vi "CheckRunProbe.vi"(0 "UiDefinition":T1) -> ()   [LabVIEW 2020]
uses:
  UIReferences.ctl
  C:/Users/User/Desktop/Automation/CurrentVersion/LabviewDXFViewer/bin/Release/LabviewDXFViewer.exe
  LabviewDXFViewer/bin/Release/LabviewDXFViewer.exe
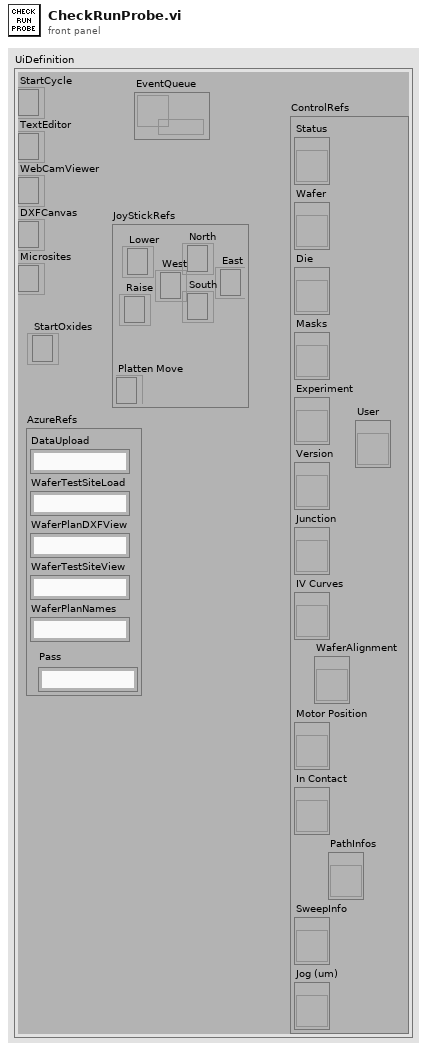
[diagram p1: front panel]
types:
  T1 = typedef "UIReferences.ctl" = cluster{"StartCycle":refnum<k24>, "TextEditor":refnum<k24>, "WebCamViewer":refnum<k24>, "DXFCanvas":refnum<k24>, "Microsites":refnum<k24>, "JoyStickRefs":cluster{"North":refnum<k24>, "Lower":refnum<k24>, "Raise":refnum<k24>, "Platten Move":refnum<k24>, "West":refnum<k24>, "East":refnum<k24>, "South":refnum<k24>}, "AzureRefs":cluster{"DataUpload":string, "WaferTestSiteLoad":string, "WaferPlanDXFView":string, "WaferTestSiteView":string, "WaferPlanNames":string, "Pass":string}, "ControlRefs":cluster{"Status":refnum<vi>, "Wafer":refnum<vi>, "Die":refnum<vi>, "Masks":refnum<vi>, "Experiment":refnum<vi>, "Version":refnum<vi>, "Junction":refnum<vi>, "IV Curves":refnum<vi>, "Motor Position":refnum<vi>, "In Contact":refnum<vi>, "SweepInfo":refnum<vi>, "Jog (um)":refnum<vi>, "PathInfos":refnum<vi>, "User":refnum<vi>, "WaferAlignment":refnum<vi>}, "EventQueue":refnum<queue>, "StartOxides":refnum<k24>}
  T2 = cluster{"Status":refnum<vi>, "Wafer":refnum<vi>, "Die":refnum<vi>, "Masks":refnum<vi>, "Experiment":refnum<vi>, "Version":refnum<vi>, "Junction":refnum<vi>, "IV Curves":refnum<vi>, "Motor Position":refnum<vi>, "In Contact":refnum<vi>, "SweepInfo":refnum<vi>, "Jog (um)":refnum<vi>, "PathInfos":refnum<vi>, "User":refnum<vi>, "WaferAlignment":refnum<vi>}
  T3 = cluster{"Die":string, "Wafer":string, "Path":path, "url":string, "Experiment":string, "Version":string, "user":string}
  T4 = typedef "WaferAlignmentType.ctl" = cluster{"Wafer Units to microns":dbl, "Rotation Misalign":dbl[], "Scale Misalign":dbl, "Steps Per micron":dbl, "Position 1":i32[], "Position 2":i32[], "Lift Distance":i32, "Position 3":i32[], "Jog Height":i32}
  T5 = cluster{"Current Range":dbl, "Source Measure Unit Channel (0: Channel A)":i32, "Waveform":waveform(dbl), "VISA resource name":refnum<visa-resource-name>, "CodeText":string}
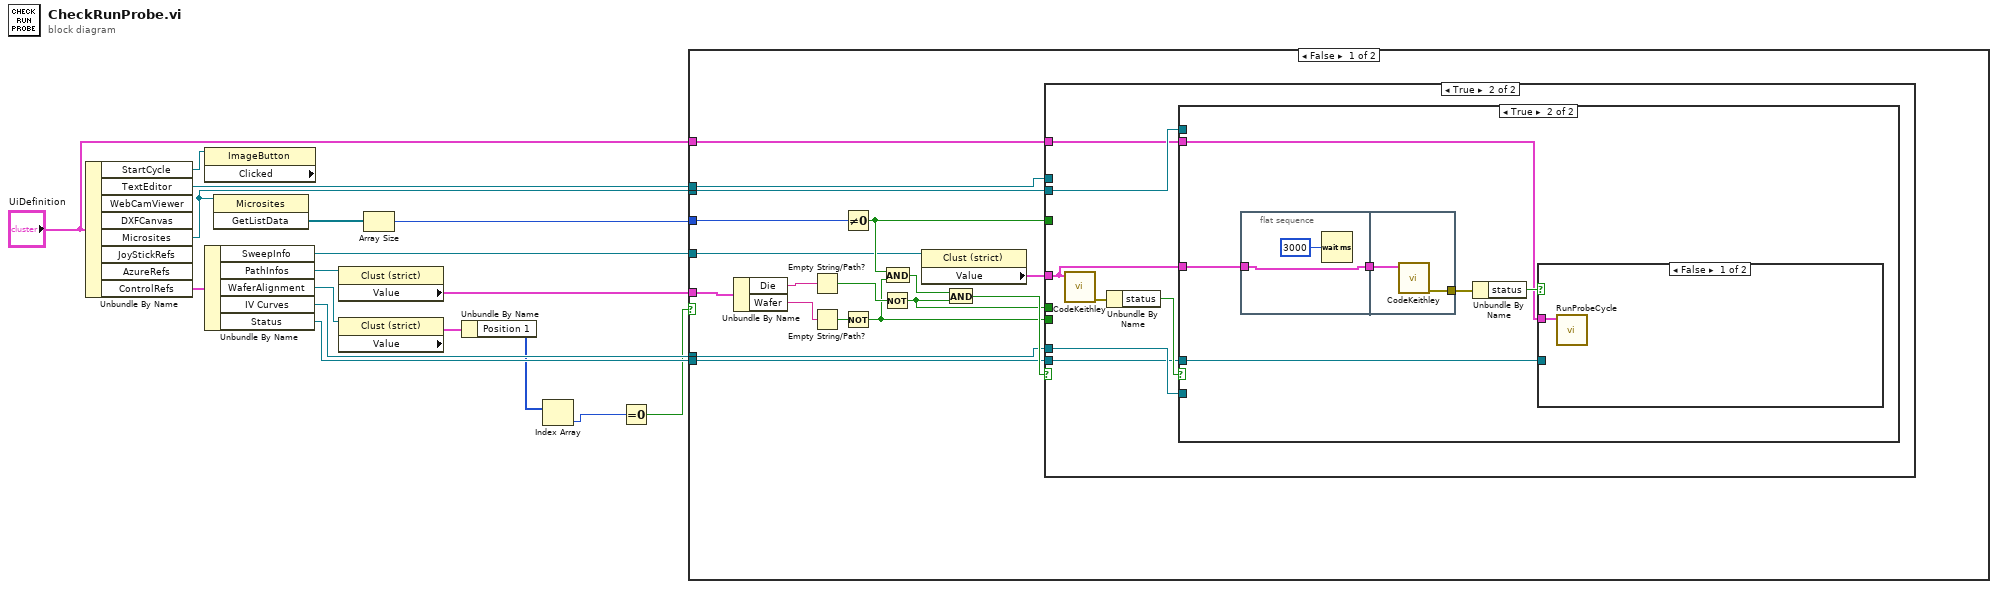
[diagram p0: block diagram]
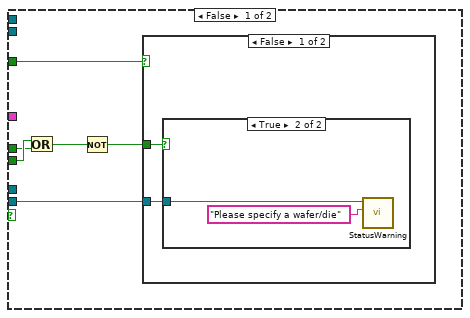
[diagram p2: hidden frame]
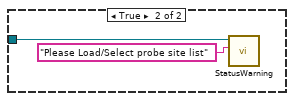
[diagram p4: hidden frame]
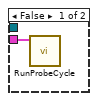
[diagram p5: hidden frame]
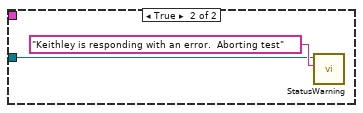
[diagram p6: hidden frame]
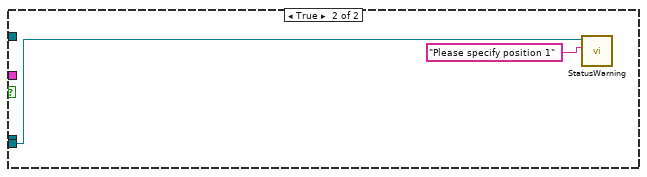
[diagram p7: hidden frame]
diagram:
  n1 = Unbundle By Name("UiDefinition") -> ("StartCycle"=w4:refnum<k24>, "TextEditor"=w8:refnum<k24>, "Microsites"=w9:refnum<k24>, "ControlRefs"=w15:T2)  [unwired: 4 out]
  n2 = property class="ImageButton" props=["Clicked"](reference=w4) -> ()  [unwired: 1 in, 3 out]
  n3 = Unbundle By Name(w15) -> ("SweepInfo"=w14:refnum<vi>, "PathInfos"=w13:refnum<vi>, "WaferAlignment"=w11:refnum<vi>, "IV Curves"=w7:refnum<vi>, "Status"=w6:refnum<vi>)
  n4 = invoke class="Microsites" method="GetListData"(reference=w9) -> ("GetListData"=w16:refnum<k24>[])  [unwired: 2 in, 2 out]
  n5 = property class="Clust (strict)"(reference=w13) -> ("Value"=w12:T3)  [unwired: 1 in, 2 out]
  n6 = property class="Clust (strict)"(reference=w11) -> ("Value"=w10:T4)  [unwired: 1 in, 2 out]
  n7 = Array Size(array=w16) -> (size(s)=w17:i32)
  n8 = Unbundle By Name(w10) -> ("Position 1"=w3:i32[])
  n9 = Index Array(array=w3) -> (element=w2:i32)  [unwired: 1 in]
  n10 = Equal To 0?(x=w2) -> (x = 0?=w1:bool)
  n11 = case shown="False" w1 {
    tunnel: w17 -> [w35 _]
    tunnel: w14 -> [w25 _]
    tunnel: w12 -> [w23 _]
    tunnel: w9 -> [w22 _]
    tunnel: w8 -> [w21 _]
    tunnel: w7 -> [w20 _]
    tunnel: w6 -> [w19 w69]
    tunnel: "UiDefinition" -> [w18 _]
    frame False {
      n12 = Unbundle By Name(w23) -> ("Die"=w26:string, "Wafer"=w27:string)
      n13 = Empty String/Path?(string/path=w26) -> (empty?=w30:bool)
      n14 = Empty String/Path?(string/path=w27) -> (empty?=w31:bool)
      n15 = Not Equal To 0?(x=w35) -> (x != 0?=w32:bool)
      n16 = Not(x=w31) -> (.not. x?=w28:bool)
      n17 = Not(x=w30) -> (.not. x?=w29:bool)
      n18 = And(x=w32, y=w28) -> (x .and. y?=w34:bool)
      n19 = property class="Clust (strict)"(reference=w25) -> ("Value"=w24:T5)  [unwired: 1 in, 2 out]
      n20 = And(x=w34, y=w29) -> (x .and. y?=w33:bool)
      n21 = case shown="True" w33 {
        tunnel: w32 -> [w41 _]
        tunnel: w28 -> [w40 _]
        tunnel: w29 -> [w39 _]
        tunnel: w21 -> [_ _]
        tunnel: w22 -> [_ w54]
        tunnel: w24 -> [_ w48]
        tunnel: w20 -> [_ w53]
        tunnel: w19 -> [w36 w50]
        tunnel: w18 -> [_ w49]
        frame False {
          n22 = Or(x=w40, y=w39) -> (x .or. y?=w38:bool)
          n23 = Not(x=w38) -> (.not. x?=w37:bool)
          n24 = case shown="False" w41 {
            tunnel: w37 -> [w43 _]
            tunnel: w36 -> [w42 w46]
            frame False {
              n25 = case shown="True" w43 {
                tunnel: w42 -> [_ w44]
                frame False {
                }
                frame True {
                  n26 = call "StatusWarning.vi"("Text.Text"="Please specify a wafer/die", "String in"=w44) -> ()  [unwired: 10 in]
                }
              }
            }
            frame True {
              n27 = call "StatusWarning.vi"("Text.Text"="Please Load/Select probe site list", "String in"=w46) -> ()  [unwired: 10 in]
            }
          }
        }
        frame True {
          n28 = call "CodeKeithley.vi"("SweepInfo"=w48) -> ("error out"=w52:errorcluster)  [unwired: 10 in]
          n29 = Unbundle By Name(w52) -> ("status"=w51:bool)
          n30 = case shown="True" w51 {
            tunnel: w54 -> [_ _]
            tunnel: w53 -> [_ _]
            tunnel: w50 -> [_ w61]
            tunnel: w49 -> [w55 w57]
            tunnel: w48 -> [_ w60]
            frame False {
              n31 = call "RunProbeCycle.vi"("UiDefinition"=w55) -> ()  [unwired: 10 in]
            }
            frame True {
              n32 = flat-sequence {
                tunnel: w60 -> [w63]
                tunnel: [w63] -> w56
                tunnel: [w64] -> w59
                tunnel: w56 -> [w65]
                frame #0 {
                  n33 = Wait (ms)(milliseconds to wait=u32 3000) -> ()  [unwired: 1 out]
                }
                frame #1 {
                  n34 = call "CodeKeithley.vi"("SweepInfo"=w65) -> ("error out"=w64:errorcluster)  [unwired: 10 in]
                }
              }
              n35 = Unbundle By Name(w59) -> ("status"=w58:bool)
              n36 = case shown="False" w58 {
                tunnel: w61 -> [_ w67]
                tunnel: w57 -> [w66 _]
                frame False {
                  n37 = call "RunProbeCycle.vi"("UiDefinition"=w66) -> ()  [unwired: 10 in]
                }
                frame True {
                  n38 = call "StatusWarning.vi"("Text.Text"="Keithley is responding with an error.  Aborting test", "String in"=w67) -> ()  [unwired: 10 in]
                }
              }
            }
          }
        }
      }
    }
    frame True {
      n39 = call "StatusWarning.vi"("Text.Text"="Please specify position 1", "String in"=w69) -> ()  [unwired: 10 in]
    }
  }
